vi "H036 Harsh Pandit SCADA Lab 5b Sem 6.vi"() -> ()   [LabVIEW 2018]
panel:
  out "Waveform Graph":dbl[](graph)
  out "Waveform Chart":dbl(graph)
  # "Experiment 5b: Create a VI to compute following expression using formula node where\ny=tanhx+cosx and where x varies from 0 to 100 in step of 0.2"
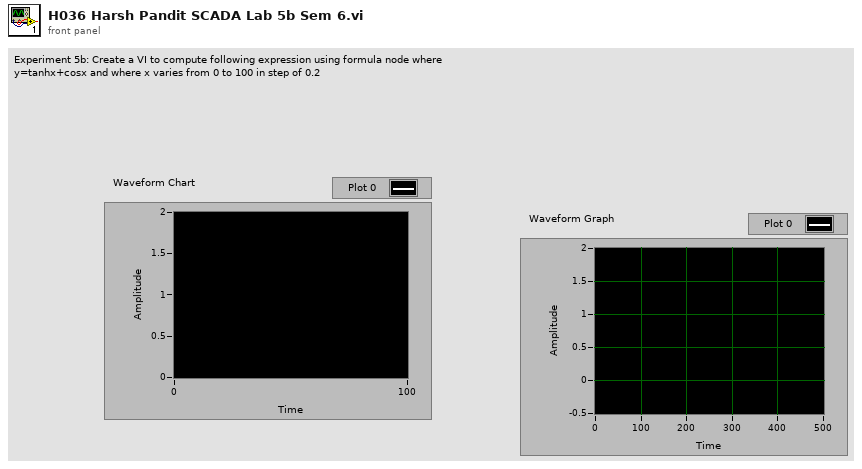
[diagram p1: front panel]
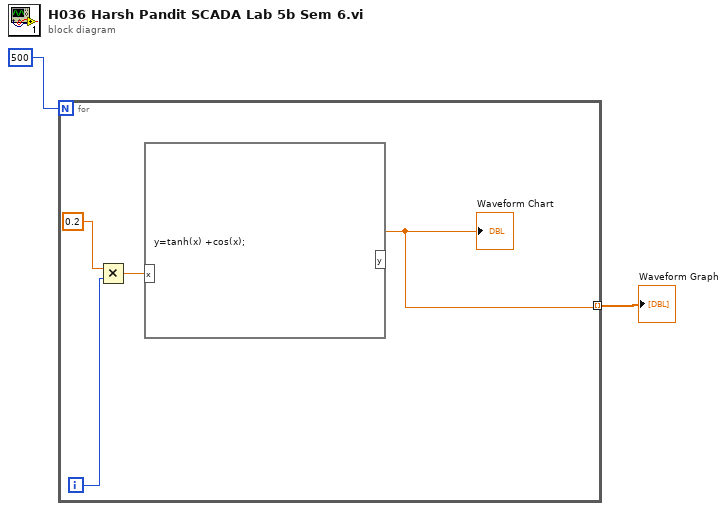
[diagram p0: block diagram]
diagram:
  n1 = for {
    N: 500 -> [_]
    tunnel: [w4] -> w1 mode=indexing
    i -> [w6]
    n2 = Multiply(x=0.2, y=w6) -> (x*y=w3:dbl)
    n3 = formula code="y=tanh(x) +cos(x);"("x"=w3) -> ("y"=w4:dbl)
    "Waveform Chart" <- w4
  }
  "Waveform Graph" <- w1
